vi "ultra.vi"() -> (3 "数值":dbl)   [LabVIEW 2015]
uses:
  <vilib>/myRIO/Instrument Drivers/Onboard IO/DIO/typedefs/DIO Reference.ctl
  <vilib>/myRIO/Common/Instrument Driver Framework/Utilities/typedefs/myRIO Generic Hardware Reference.ctl
  <vilib>/myRIO/Common/Instrument Driver Framework/Utilities/typedefs/Hardware Version Enum.ctl
  <vilib>/myRIO/Common/Instrument Driver Framework/Utilities/typedefs/myRIO v1.0 Reference.ctl
  <vilib>/myRIO/Common/Instrument Driver Framework/Utilities/typedefs/Generic FPGA Reference.ctl
  <vilib>/myRIO/Common/Instrument Driver Framework/myRIO v1.0/DIO/typedefs/DIO Channels List.ctl
  <vilib>/myRIO/Common/Instrument Driver Framework/myRIO v1.0/DIO/typedefs/DIO Channels Enum.ctl
  <vilib>/userdefined/High Color/nirio_resource_hc.ctl
  <vilib>/myRIO/Common/Instrument Driver Framework/Utilities/vis/Is FPGA Ref Available.vi
  <vilib>/myRIO/Common/Instrument Driver Framework/myRIO v1.0/DIO/vis/myRIO v1.1 Open DIO.vi
  <vilib>/myRIO/Instrument Drivers/Onboard IO/DIO/vis/Write.vi
  <vilib>/myRIO/Instrument Drivers/Onboard IO/DIO/vis/Read.vi
  <vilib>/myRIO/Common/Instrument Driver Framework/Utilities/vis/Validate Channels.vi
  <vilib>/myRIO/Common/Instrument Driver Framework/myRIO v1.0/DIO/vis/myRIO v1.0 Reserve DIO.vi
  <vilib>/myRIO/Common/Instrument Driver Framework/myRIO v1.0/Resource Manager/vis/myRIO v1.0 Reserve Channel List.vi
  <vilib>/myRIO/Common/Instrument Driver Framework/myRIO v1.0/DIO/vis/myRIO v1.0 Build MUX Configuration DIO.vi
  <vilib>/myRIO/Common/Instrument Driver Framework/myRIO v1.0/Resource Manager/vis/myRIO v1.0 Reserve Channel.vi
  <vilib>/myRIO/Common/Instrument Driver Framework/myRIO v1.0/Resource Manager/vis/myRIO v1.0 Unreserve Channel.vi
  <vilib>/myRIO/Common/Instrument Driver Framework/myRIO v1.0/Resource Manager/vis/myRIO v1.0 Create Configuration List.vi
  <vilib>/myRIO/Common/Instrument Driver Framework/myRIO v1.0/Resource Manager/vis/myRIO v1.0 Build Mutex Name.vi
  <vilib>/Utility/VariantDataType/GetNumericInfo.vi
  <vilib>/Utility/error.llb/Error Cluster From Error Code.vi
  <vilib>/myRIO/Common/Instrument Driver Framework/myRIO v1.0/myRIO v1.1 Open.vi
  <vilib>/myRIO/Common/Instrument Driver Framework/Utilities/vis/IO Manager.vi
  <vilib>/myRIO/Common/Instrument Driver Framework/Utilities/vis/Configuration Manager.vi
  <vilib>/myRIO/Common/Instrument Driver Framework/myRIO v1.0/Resource Manager/vis/myRIO v1.0 Configure IO.vi
  <vilib>/myRIO/Common/Instrument Driver Framework/myRIO v1.0/myRIO v1.0 Close.vi
  <vilib>/myRIO/Common/Instrument Driver Framework/myRIO v1.0/DIO/vis/myRIO v1.0 Write DIO.vi
  <vilib>/myRIO/Common/Instrument Driver Framework/myRIO v1.0/DIO/vis/myRIO v1.0 Read DIO.vi
  <vilib>/myRIO/Express VI/Onboard IO/DO/DO Express VI.xnode
  <vilib>/myRIO/Instrument Drivers/Onboard IO/DIO/vis/myRIO DIO Open.xnode
  <vilib>/myRIO/Express VI/Onboard IO/DI/DI Express VI.xnode
  <vilib>/myRIO/Instrument Drivers/Onboard IO/DIO/DIO.lvlib
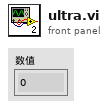
[diagram p1: front panel]
types:
  T1 = typedef "DIO.lvlib/DIO Reference.ctl" = cluster{"myRIO Reference":T2, "DIO Channels List":T6}
  T2 = typedef "myRIO Generic Hardware Reference.ctl" = cluster{"myRIO Model":T3, "myRIO Hardware Reference":T4}
  T3 = typedef "Hardware Version Enum.ctl" = enum16{"Unknown", "myRIO-1900", "myRIO-1950", "roboRIO"}
  T4 = typedef "myRIO v1.0 Reference.ctl" = cluster{"Generic FPGA Reference":T5, "Allow multiple opens":bool}
  T5 = typedef "Generic FPGA Reference.ctl" = refnum<k20>
  T6 = typedef "DIO Channels List.ctl" = T7[]
  T7 = typedef "DIO Channels Enum.ctl" = enum16{"Not Connected", "C/DIO0", "C/DIO1", "C/DIO2", "C/DIO3", "C/DIO4", "C/DIO5", "C/DIO6", "C/DIO7", "A/DIO0", "A/DIO1", "A/DIO2", "A/DIO3", "A/DIO4", "A/DIO5", "A/DIO6", "A/DIO7", "A/DIO8", "A/DIO9", "A/DIO10", "A/DIO11", "A/DIO12", "A/DIO13", "A/DIO14", "A/DIO15", "B/DIO0", "B/DIO1", "B/DIO2", "B/DIO3", "B/DIO4", "B/DIO5", "B/DIO6", "B/DIO7", "B/DIO8", "B/DIO9", "B/DIO10", "B/DIO11", "B/DIO12", "B/DIO13", "B/DIO14", "B/DIO15", "LED0", "LED1", "LED2", "LED3", "Button0", "DIO/DIO0", "DIO/DIO1", "DIO/DIO2", "DIO/DIO3", "DIO/DIO4", "DIO/DIO5", "DIO/DIO6", "DIO/DIO7", "DIO/DIO8", "DIO/DIO9", "SPI/CS0", "SPI/CS1", "SPI/CS2", "SPI/CS3", "LED RADIO (Green)", "LED RADIO (Red)", "LED COMM (Green)", "LED COMM (Red)", "LED MODE (Green)", "LED MODE (Red)"}
  T8 = typedef "nirio_resource_hc.ctl" = tag
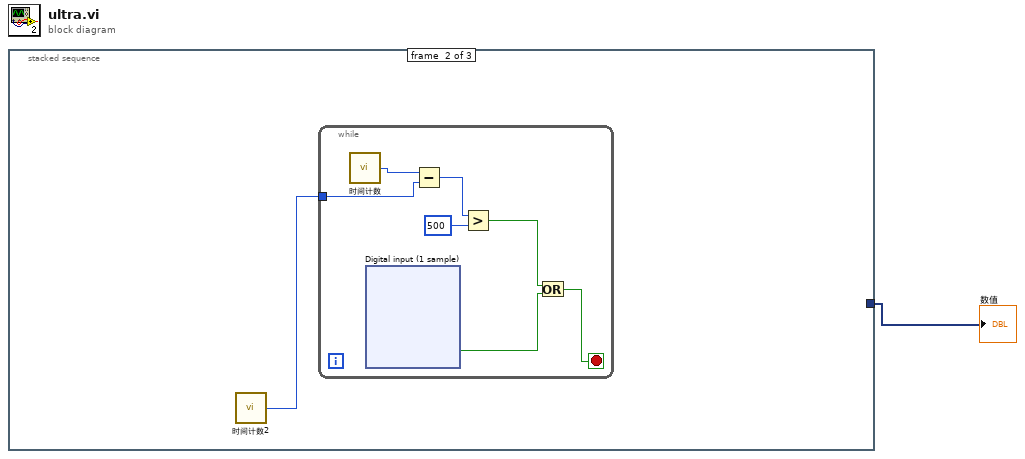
[diagram p0: block diagram]
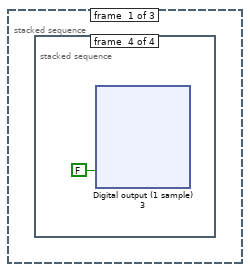
[diagram p2: hidden frame]
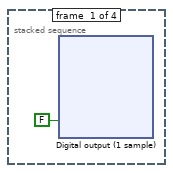
[diagram p3: hidden frame]
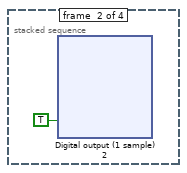
[diagram p4: hidden frame]
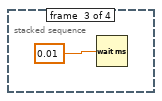
[diagram p5: hidden frame]
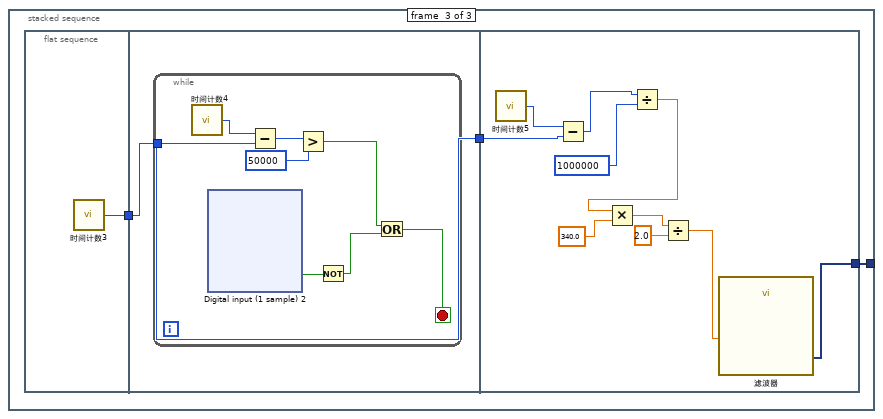
[diagram p6: hidden frame]
diagram:
  n1 = stacked-sequence {
    tunnel: [_ _ w154] -> w1
    frame #0 {
      n2 = stacked-sequence {
        frame #0 {
          n3 = xnode "Digital output (1 sample)"("A/DIO10 (Pin 31)"=FALSE) -> ()  [unwired: 1 in, 1 out]
        }
        frame #1 {
          n4 = xnode "Digital output (1 sample) 2"("A/DIO10 (Pin 31)"=TRUE) -> ()  [unwired: 1 in, 1 out]
        }
        frame #2 {
          n5 = Wait (ms)(milliseconds to wait=0.01 ("等待时间（毫秒）")) -> ()  [unwired: 1 out]
        }
        frame #3 {
          n6 = xnode "Digital output (1 sample) 3"("A/DIO10 (Pin 31)"=FALSE) -> ()  [unwired: 1 in, 1 out]
        }
      }
    }
    frame #1 {
      n7 = call "时间计数2"() -> ("Tick Count(uSec)"=w111:u32)
      n8 = while {
        tunnel: w111 -> [w117]
        stop <- w112 stop-if-true
        n9 = call "时间计数"() -> ("Tick Count(uSec)"=w118:u32)
        n10 = xnode "Digital input (1 sample)"() -> ("A/DIO7 (Pin 25)"=w114:bool)  [unwired: 1 in, 1 out]
        n11 = Subtract(x=w118, y=w117) -> (x-y=w116:u32)
        n12 = Greater?(x=w116, y=u32 500) -> (0:w113:bool)
        n13 = Or(x=w113, y=w114) -> (x .or. y?=w112:bool)
      }
    }
    frame #2 {
      n14 = flat-sequence {
        tunnel: [w157] -> w156
        tunnel: w156 -> [w158]
        tunnel: [w158] -> w155
        tunnel: w155 -> [w210]
        tunnel: [w202] -> w154
        frame #0 {
          n15 = call "时间计数3"() -> ("Tick Count(uSec)"=w157:u32)
        }
        frame #1 {
          n16 = while {
            tunnel: w158 -> [w165]
            stop <- w159 stop-if-true
            n17 = call "时间计数4"() -> ("Tick Count(uSec)"=w166:u32)
            n18 = xnode "Digital input (1 sample) 2"() -> ("A/DIO7 (Pin 25)"=w162:bool)  [unwired: 1 in, 1 out]
            n19 = Subtract(x=w166, y=w165) -> (x-y=w164:u32)
            n20 = Greater?(x=w164, y=u32 50000) -> (0:w161:bool)
            n21 = Not(x=w162) -> (.not. x?=w160:bool)
            n22 = Or(x=w161, y=w160) -> (x .or. y?=w159:bool)
          }
        }
        frame #2 {
          n23 = call "时间计数5"() -> ("Tick Count(uSec)"=w211:u32)
          n24 = Subtract(x=w211, y=w210) -> (x-y=w209:u32)
          n25 = Divide(x=w209, y=u32 1000000) -> (x/y=w205:dbl)
          n26 = Multiply(x=w205, y=340.0) -> (x*y=w206:dbl)
          n27 = Divide(x=w206, y=2.0) -> (x/y=w203:dbl)
          n28 = call "滤波器"("Signal"=w203) -> ("Filtered Signal"=w202:dynamicdata)  [unwired: 9 in, 1 out]
        }
      }
    }
  }
  "数值" <- w1
